vi "Main_PhaseShifting.vi"() -> ()   [LabVIEW 2020]
uses:
  Controls/Control_Camara.ctl
  <vilib>/userdefined/High Color/IMAQdx.ctl
  Controls/Control_MaquinaEstados.ctl
  Controls/Control_RegistroDeDatos.ctl
  <vilib>/vision/Image Controls.llb/IMAQ Image.ctl
  <vilib>/Instr/_visa.llb/VISA Find Search Mode.ctl
  <vilib>/Instr/_visa.llb/VISA Configure Serial Port (Instr).vi
  <vilib>/vision/driver/NI_Vision_Acquisition_Software.lvlib
panel:
  in  "Session In":T1
  out "InterfaceName":string
  in  "Numero de Pasos":i32=5
  in  "Delay piezoeléctrico (ms)":u32=500
  in  "Nombre de la Imagen":string="Referencia"
  out "Voltaje Enviado":string[](array[string])
  in  "SnapShot":bool
  out "Pantalla":T2(plugin-control)
  in  "Puerto":refnum<visa-resource-name>="COM2"
  in  "Fotos":T3
  in  "Calibrar":bool
  in  "stop":bool
  # "#TODO: add selector for manual/auto phase shifting."
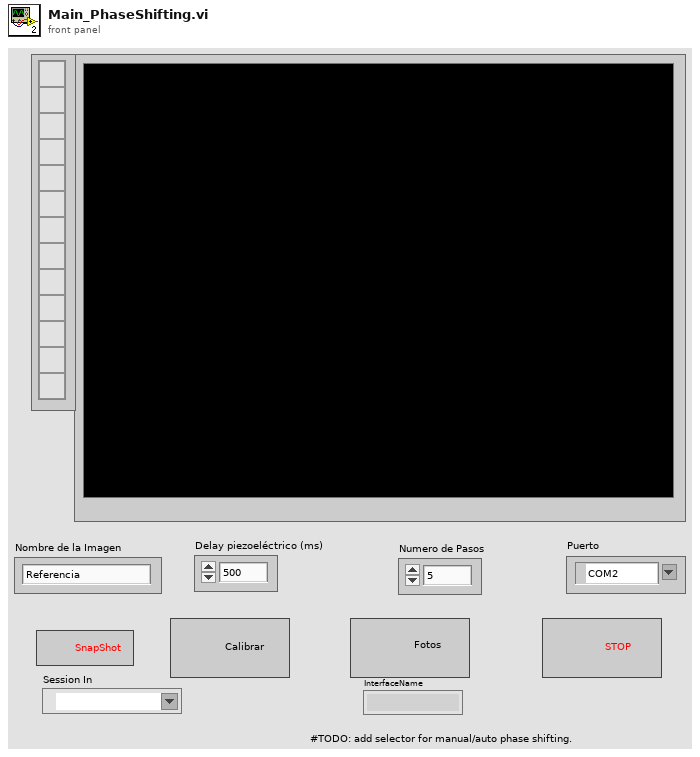
[diagram p1: front panel]
types:
  T1 = typedef "IMAQdx.ctl" = refnum<k21>
  T2 = typedef "IMAQ Image.ctl" = refnum<image>
  T3 = typedef "Control_Camara.ctl" = bool
  T4 = typedef "Control_RegistroDeDatos.ctl" = cluster{"V 2Pi Actual":sgl, "Puerto":refnum<visa-resource-name>, "InterfaceName":string, "Canal":string, "dt (ms)":u16, "Referencias":cluster{"Calibrar":refnum<vi>, "Fotos":refnum<vi>, "stop":refnum<vi>, "SnapShot":refnum<vi>}, "Imagenes":T2[], "Session Out":T1, "Bandera":bool}
  T5 = typedef "Control_MaquinaEstados.ctl" = enum16{"Esperar", "Inicializar", "Calibración", "Fotos", "Grabando", "Inicializar dispositivos", "Fase", "Cerrar dispositivos", "Exit"}
  T6 = typedef "VISA Find Search Mode.ctl" = u32
  T7 = cluster{"Type":u32, "Version":u32, "Flags":u32, "SerialNumberHigh":u32, "SerialNumberLow":u32, "BusType":u32, "InterfaceName":string, "VendorName":string, "ModelName":string, "CameraFileName":string, "CameraAttributeURL":string}[]
  T8 = cluster{"Type":u32, "Version":u32, "Flags":u32, "SerialNumberHigh":u32, "SerialNumberLow":u32, "BusType":u32, "InterfaceName":string, "VendorName":string, "ModelName":string, "CameraFileName":string, "CameraAttributeURL":string}
  T9 = cluster{"Calibrar":refnum<vi>, "Fotos":refnum<vi>, "stop":refnum<vi>, "SnapShot":refnum<vi>}
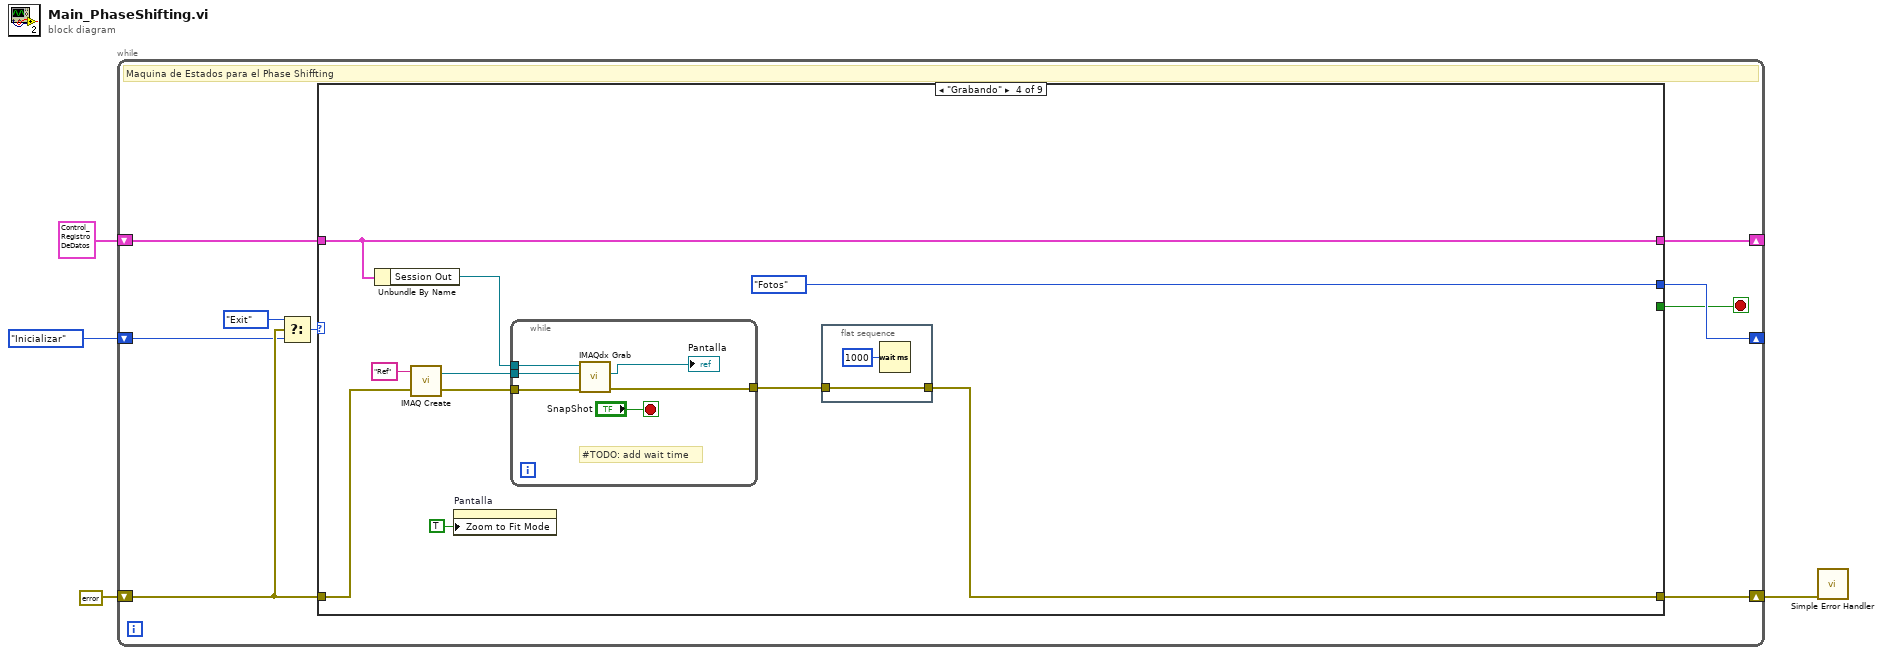
[diagram p0: block diagram]
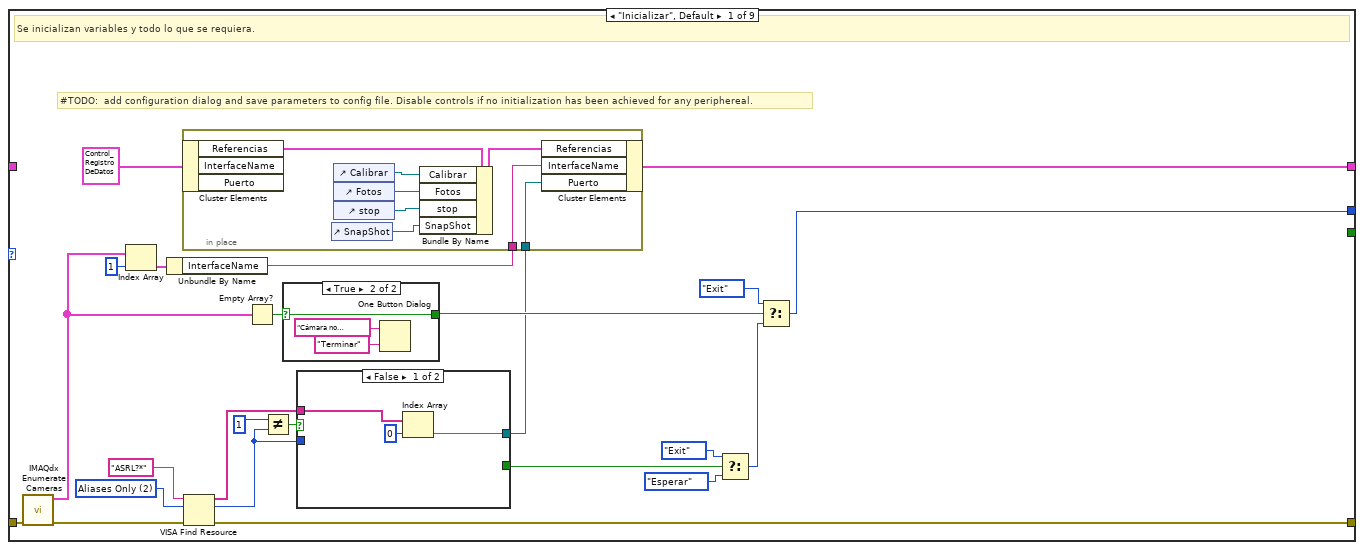
[diagram p2: hidden frame]
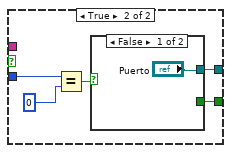
[diagram p3: hidden frame]
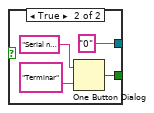
[diagram p4: hidden frame]
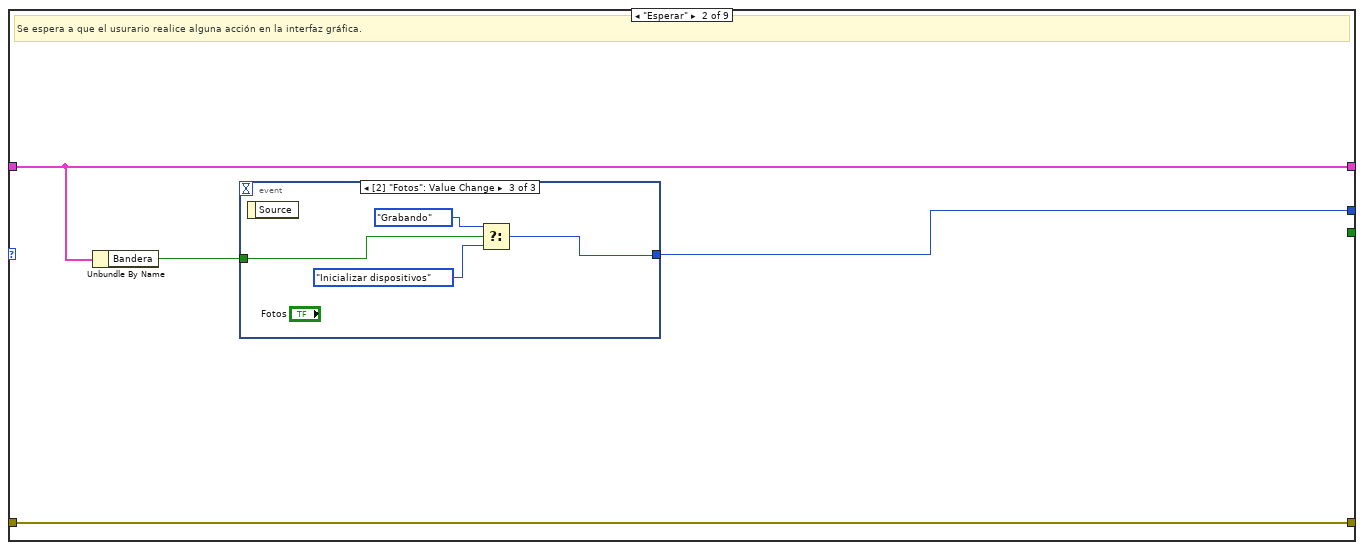
[diagram p6: hidden frame]
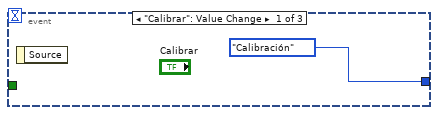
[diagram p7: hidden frame]
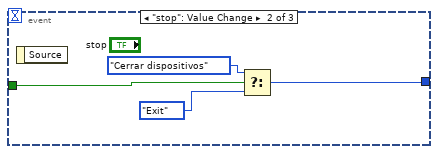
[diagram p8: hidden frame]
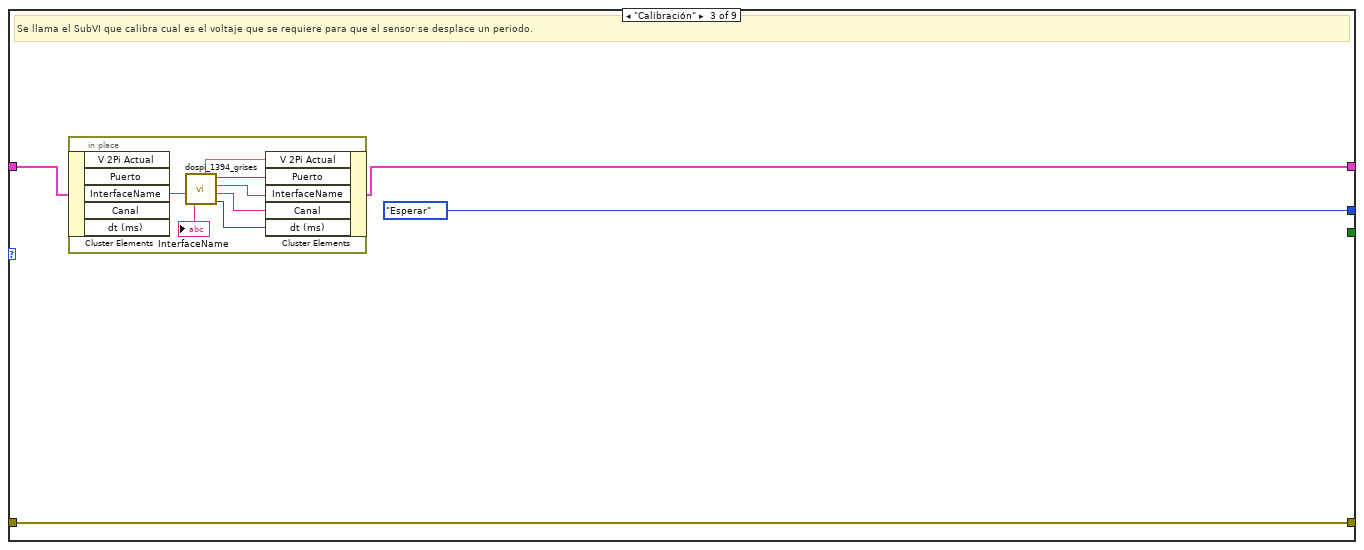
[diagram p9: hidden frame]
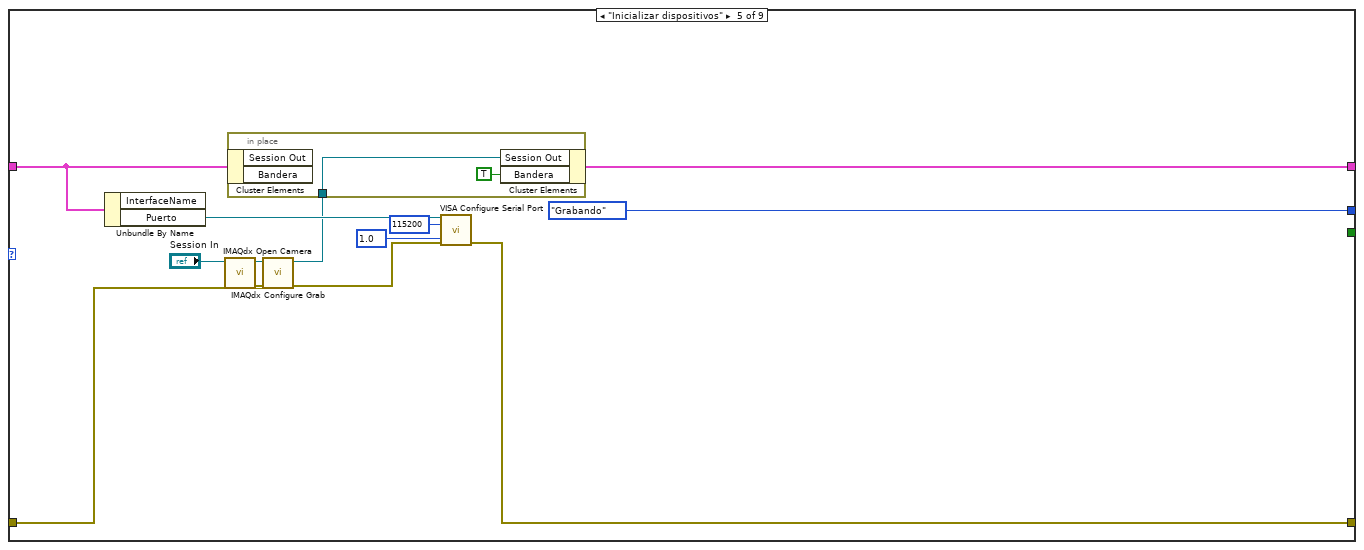
[diagram p10: hidden frame]
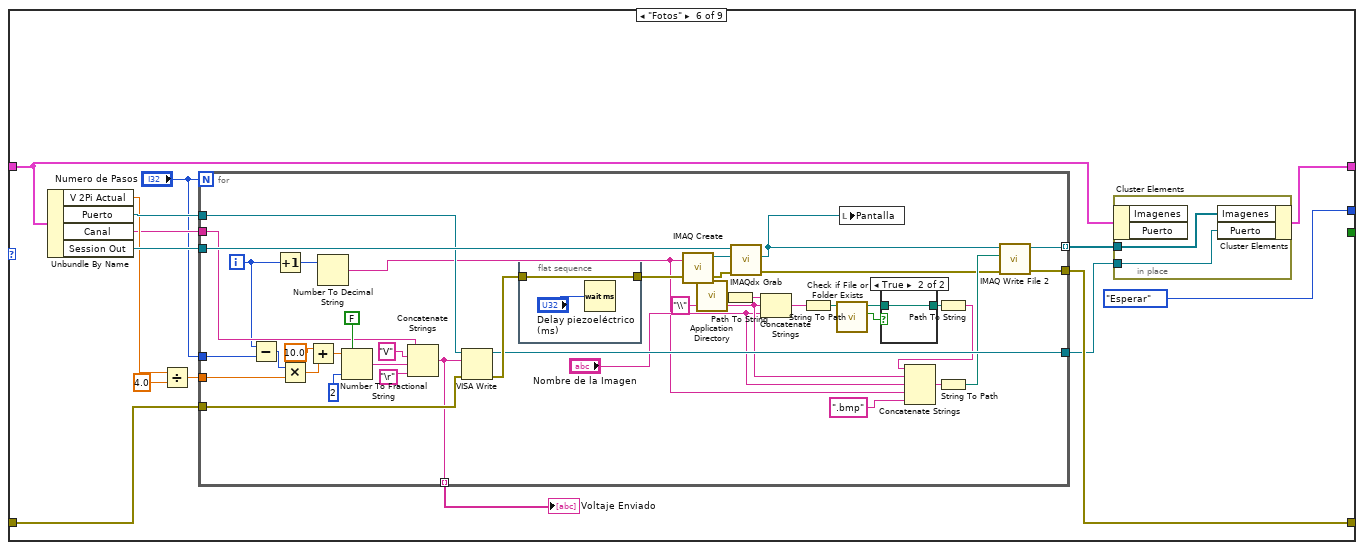
[diagram p11: hidden frame]
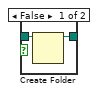
[diagram p12: hidden frame]
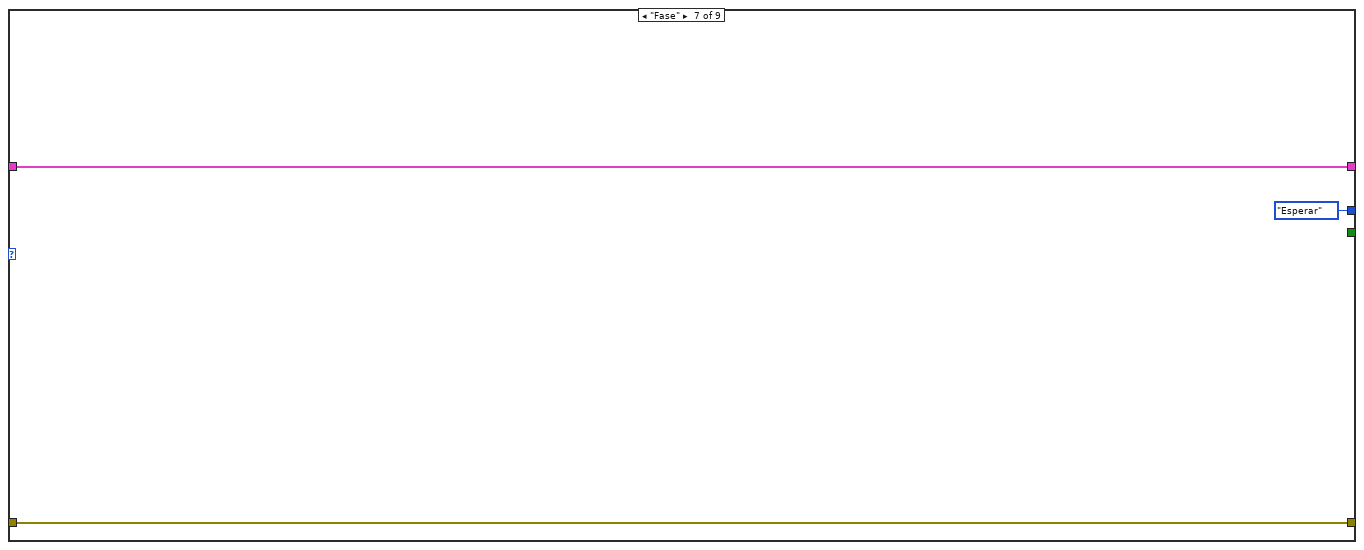
[diagram p13: hidden frame]
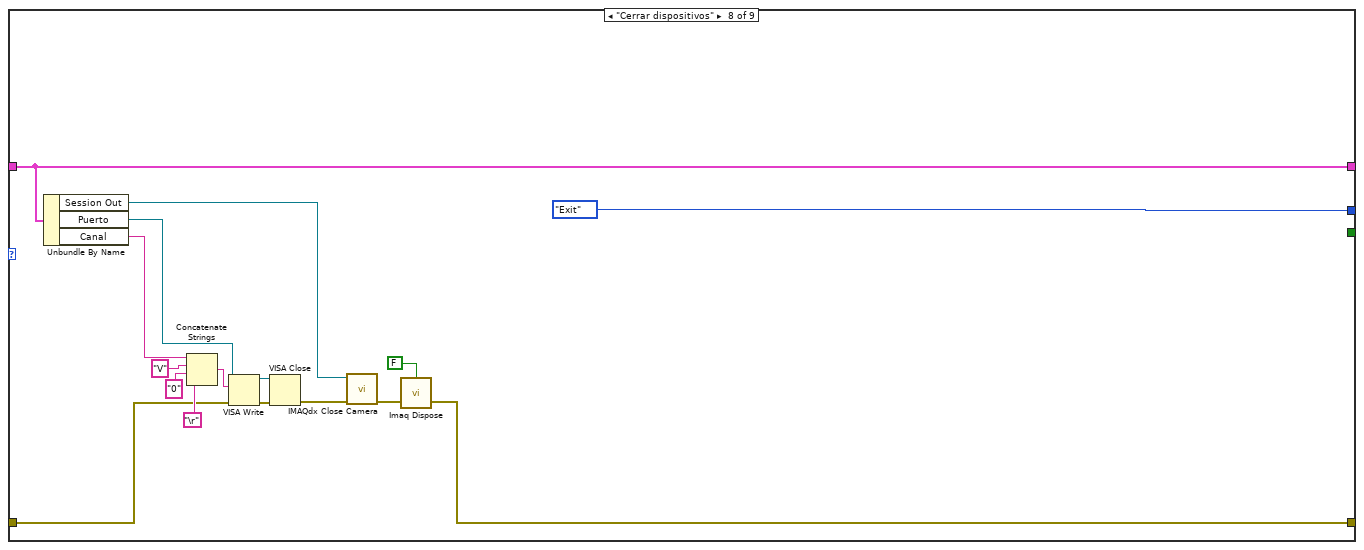
[diagram p14: hidden frame]
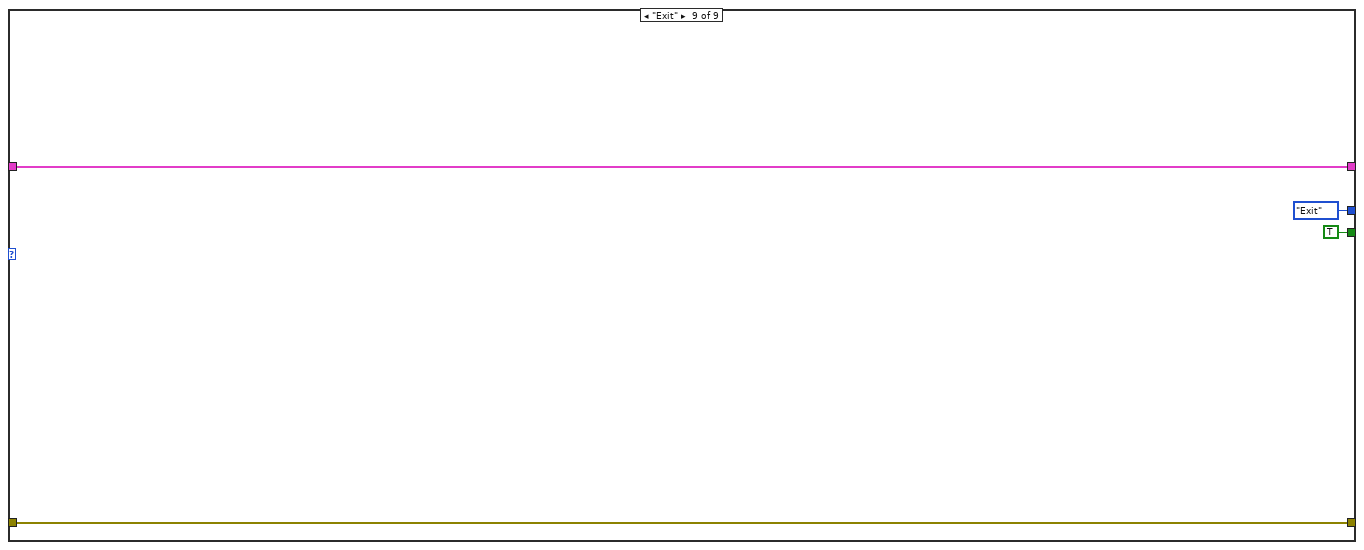
[diagram p15: hidden frame]
diagram:
  n1 = while {
    shift-right: [w13] -> _
    shift-left: Control_MaquinaEstados."Inicializar" ("Enum") -> [w10]
    shift-right: [w12] -> _
    shift-left: T4 {"V 2Pi Actual"=0.0, "Puerto"="COM3", "InterfaceName"="", "Canal"="", "dt (ms)"=0, "Referencias"={"Calibrar"=refnum, "Fotos"=refnum, "stop"=refnum, "SnapShot"=refnum}, "Imagenes"=[], "Session Out"="cam11", "Bandera"=FALSE} -> [w5]
    shift-right: [w6] -> w3
    shift-left: errorcluster {"status"=FALSE, "code"=0, "source"=""} ("Error In") -> [w11]
    stop <- w7 stop-if-true
    # "Maquina de Estados para el Phase Shiffting"
    n2 = Select(t=Control_MaquinaEstados."Exit", s=w11, f=w10) -> (s? t:f=w8:T5)
    n3 = case shown="\"Grabando\"" w8 {
      tunnel: [w19 w66 Control_MaquinaEstados."Esperar" ("Enum") Control_MaquinaEstados."Fotos" ("Enum") Control_MaquinaEstados."Grabando" ("Enum") Control_MaquinaEstados."Esperar" ("Enum") Control_MaquinaEstados."Esperar" ("Enum") Control_MaquinaEstados."Exit" ("Enum") Control_MaquinaEstados."Exit" ("Enum")] -> w13
      tunnel: w5 -> [_ w64 w79 w88 w107 w126 w184 w193 w204]
      tunnel: [w37 w64 w78 w88 w105 w123 w184 w193 w204] -> w12
      tunnel: [_ _ _ _ _ _ _ _ TRUE] -> w7
      tunnel: w11 -> [w17 w65 w76 w94 w109 w132 w183 w190 w203]
      tunnel: [w15 w65 w76 w89 w112 w131 w183 w185 w203] -> w6
      frame "Inicializar", Default {
        w31 = T6 2 items=["Canonical Names Only"=0, "Aliases Only"=2, "Include Matching Aliases"=3, "Include All Aliases"=4] ("Search Mode")
        # "#TODO:  add configuration dialog and save parameters to config file. Disable controls if no initialization has been achieved for any periphereal."
        # "Se inicializan variables y todo lo que se requiera."
        n4 = call <vilib>:"IMAQdx Enumerate Cameras.vi"("error in"=w17) -> ("error out"=w16:errorcluster, "Camera Information Array"=w29:T7)  [unwired: 9 in]
        n5 = Index Array(array=w29, index=1) -> (element=w28:T8)
        n6 = Unbundle By Name(w28) -> ("InterfaceName"=w26:string)
        n7 = VISA Find Resource(8:w16, 10:w31, 11:"ASRL?*" ("expression (\"?*\")")) -> (0:w15:errorcluster, 2:w35:u32, 3:w34:string[])
        n8 = Empty Array?(array=w29) -> (empty?=w30:bool)
        n9 = Not Equal?(x=u32 1 ("y"), y=w35) -> (x != y?=w33:bool)
        n10 = case shown="True" w30 {
          selector: w30 -> [w51 w52]
          tunnel: [w51 w52] -> w25
          frame False {
          }
          frame True {
            n11 = One Button Dialog(message="Cámara no encontrada" ("error source (\" \")"), button name ("OK")="Terminar") -> ()  [unwired: 1 out]
          }
        }
        n12 = case shown="False" w33 {
          tunnel: w34 -> [w40 _]
          tunnel: [w38 w45] -> w18
          tunnel: w35 -> [_ w44]
          tunnel: [_ w42] -> w24
          frame False {
            n13 = Index Array(array=w40, index=0) -> (element=w38:string)
          }
          frame True {
            n14 = Equal?(x=w44, y=u32 0) -> (x = y?=w43:bool)
            n15 = case shown="False" w43 {
              tunnel: ["Puerto" "0" ("button name (\"OK\")")] -> w45
              tunnel: [_ w48] -> w42
              frame False {
              }
              frame True {
                n16 = One Button Dialog(message="Serial no encontrado" ("error source (\" \")"), button name ("OK")="Terminar") -> (true=w48:bool)
              }
            }
          }
        }
        n17 = in-place {
          in-place-border: w26 -> [w57]
          in-place-border: w18 -> [w56]
          n18 = in-place-cluster #1(T4 {"V 2Pi Actual"=0.0, "Puerto"="COM3", "InterfaceName"="", "Canal"="", "dt (ms)"=0, "Referencias"={"Calibrar"=refnum, "Fotos"=refnum, "stop"=refnum, "SnapShot"=refnum}, "Imagenes"=[], "Session Out"="cam11", "Bandera"=FALSE}) -> ("Referencias"=w62:T9)  [unwired: 2 out]
          n19 = control-ref of="SnapShot"() -> (w55:refnum<vi>)
          n20 = control-ref of="Calibrar"() -> (w60:refnum<vi>)
          n21 = control-ref of="Fotos"() -> (w59:refnum<vi>)
          n22 = control-ref of="stop"() -> (w58:refnum<vi>)
          n23 = Bundle By Name(cluster=w62, "Calibrar"=w60, "Fotos"=w59, "stop"=w58, "SnapShot"=w55) -> (w61:T9)
          n24 = in-place-cluster #1("Referencias"=w61, "InterfaceName"=w57, "Puerto"=w56) -> (w37:T4)
        }
        n25 = Select(t=Control_MaquinaEstados."Exit" ("Enum"), s=w24, f=Control_MaquinaEstados."Esperar" ("Enum")) -> (s? t:f=w21:T5)
        n26 = Select(t=Control_MaquinaEstados."Exit" ("Enum"), s=w25, f=w21) -> (s? t:f=w19:T5)
      }
      frame "Esperar" {
        # "Se espera a que el usurario realice alguna acción en la interfaz gráfica."
        n27 = Unbundle By Name(w64) -> ("Bandera"=w63:bool)
        n28 = event shown="[2] \"Fotos\": Value Change" {
          selector: _ -> [_ _ _]
          dyn-events: _ -> [_ _ _]
          timeout: _ -> [_ _ _]
          tunnel: [Control_MaquinaEstados."Calibración" ("Enum") w68 w73] -> w66
          tunnel: w63 -> [_ w71 w75]
          event "Calibrar": Value Change {
            n29 = event-data() -> ()  [unwired: 1 in, 1 out]
          }
          event "stop": Value Change {
            n30 = event-data() -> ()  [unwired: 1 in, 1 out]
            n31 = Select(t=Control_MaquinaEstados."Cerrar dispositivos" ("Enum"), s=w71, f=Control_MaquinaEstados."Exit" ("Enum")) -> (s? t:f=w68:T5)
          }
          event Value Change {
            n32 = event-data() -> ()  [unwired: 1 in, 1 out]
            n33 = Select(t=Control_MaquinaEstados."Grabando" ("Enum"), s=w75, f=Control_MaquinaEstados."Inicializar dispositivos" ("Enum")) -> (s? t:f=w73:T5)
          }
        }
      }
      frame "Calibración" {
        # "Se llama el SubVI que calibra cual es el voltaje que se requiere para que el sensor se desplace un periodo."
        n34 = in-place {
          n35 = in-place-cluster #2(w79) -> ("InterfaceName"=→"InterfaceName":string)  [unwired: 4 out]
          n36 = call "dospi_1394_grises.vi"() -> ("dt (ms) 2"=w81:u16, "Canal 2"=w82:string, "InterfaceName"=w83:string, "Puerto 2"=w84:refnum<visa-resource-name>, "V 2Pi\nActual"=w85:sgl)  [unwired: 6 in, 1 out]
          n37 = in-place-cluster #2("V 2Pi Actual"=w85, "Puerto"=w84, "InterfaceName"=w83, "Canal"=w82, "dt (ms)"=w81) -> (w78:T4)
        }
      }
      frame "Grabando" {
        n38 = Unbundle By Name(w88) -> ("Session Out"=w87:T1)
        n39 = call "IMAQ Create"("Image Name"="Ref", "error in (no error)"=w94) -> ("New Image"=w93:T2, "error out"=w91:errorcluster)  [unwired: 3 in]
        n40 = property on="Pantalla" class="ImageControl"("Zoom to Fit Mode"=TRUE) -> ()  [unwired: 2 in, 2 out]
        n41 = while {
          tunnel: w87 -> [w103]
          tunnel: w91 -> [w102]
          tunnel: w93 -> [w101]
          tunnel: [w98] -> w90
          stop <- "SnapShot" stop-if-true
          # "#TODO: add wait time"
          n42 = call <vilib>:"IMAQdx Grab.vi"("error in"=w102, "Image In"=w101, "Session In"=w103) -> ("error out"=w98:errorcluster, "Image Out"=→"Pantalla":T2)  [unwired: 5 in, 2 out]
        }
        n43 = flat-sequence {
          tunnel: w90 -> [w96]
          tunnel: [w96] -> w89
          frame #0 {
            n44 = Wait (ms)(milliseconds to wait=u32 1000) -> ()  [unwired: 1 out]
          }
        }
      }
      frame "Inicializar dispositivos" {
        w114 = u16 10 items=["1.0"=10, "1.5"=15, "2.0"=20] ("stop bits (10: 1 bit)")
        n45 = Unbundle By Name(w107) -> ("Puerto"=w111:refnum<visa-resource-name>)  [unwired: 1 out]
        n46 = call <vilib>:"IMAQdx Open Camera.vi"("error in"=w109, "Session In"="Session In") -> ("error out"=w115:errorcluster, "Session Out"=w116:T1)  [unwired: 8 in]
        n47 = call <vilib>:"IMAQdx Configure Grab.vi"("error in"=w115, "Session In"=w116) -> ("error out"=w108:errorcluster, "Session Out"=w106:T1)  [unwired: 8 in]
        n48 = in-place {
          in-place-border: w106 -> [w118]
          n49 = in-place-cluster #3(w107) -> ()  [unwired: 2 out]
          n50 = in-place-cluster #3("Session Out"=w118, "Bandera"=TRUE) -> (w105:T4)
        }
        n51 = call-poly "VISA Configure Serial Port"("VISA resource name"=w111, "baud rate (9600)"=u32 115200, "error in (no error)"=w108, "stop bits (10: 1 bit)"=w114) -> ("error out"=w112:errorcluster)  [unwired: 10 in, 1 out]
      }
      frame "Fotos" {
        n52 = Unbundle By Name(w126) -> ("V 2Pi Actual"=w129:sgl, "Puerto"=w130:refnum<visa-resource-name>, "Canal"=w127:string, "Session Out"=w133:T1)
        n53 = Divide(x=w129, y=sgl 4.0) -> (x/y=w128:sgl)
        n54 = for {
          N: "Numero de Pasos" -> [_]
          tunnel: w133 -> [w176]
          tunnel: w132 -> [w160]
          tunnel: [w153] -> w125 mode=indexing
          tunnel: [w154] -> w131
          tunnel: w130 -> [w165]
          tunnel: w128 -> [w161]
          tunnel: w127 -> [w164]
          tunnel: [w156] -> w124
          tunnel: [w155] -> w120 mode=indexing
          tunnel: "Numero de Pasos" -> [w136]
          i -> [w162]
          w143 = "\\" ("string")
          n55 = Subtract(x=w162, y=w136) -> (x-y=w163:i32)
          n56 = Increment(x=w162) -> (x+1=w175:i32)
          n57 = Multiply(x=w163, y=w161) -> (x*y=w166:sgl)
          n58 = Add(x=sgl 10.0, y=w166) -> (x+y=w173:sgl)
          n59 = Number To Decimal String(number=w175) -> (decimal integer string=w141:string)  [unwired: 1 in]
          n60 = Number To Fractional String(use system decimal point (T)=FALSE, number=w173, precision (6)=i16 2) -> (F-format string=w167:string)  [unwired: 1 in]
          n61 = Concatenate Strings(w164, "V" ("Substring"), w167, "\r") -> (w155:string)
          n62 = VISA Write(VISA resource name=w165, write buffer=w155, error in (no error)=w160) -> (VISA resource name out=w156:refnum<visa-resource-name>, error out=w158:errorcluster)  [unwired: 1 out]
          n63 = flat-sequence {
            tunnel: w158 -> [w180]
            tunnel: [w180] -> w157
            frame #0 {
              n64 = Wait (ms)(milliseconds to wait="Delay piezoeléctrico (ms)") -> ()  [unwired: 1 out]
            }
          }
          n65 = call "IMAQ Create"("Image Name"=w141, "error in (no error)"=w157) -> ("New Image"=w174:T2, "error out"=w159:errorcluster)  [unwired: 3 in]
          n66 = call <vilib>:"Application Directory.vi"() -> ("Application Directory"=w152:path)
          n67 = Path To String(path=w152) -> (string=w151:string)
          n68 = call <vilib>:"IMAQdx Grab.vi"("error in"=w159, "Image In"=w174, "Session In"=w176) -> ("error out"=w138:errorcluster, "Image Out"=w137:T2)  [unwired: 5 in, 2 out]
          n69 = Concatenate Strings(w151, w143, "Nombre de la Imagen") -> (w150:string)
          n70 = String To Path(string=w150) -> (path=w147:path)
          n71 = call <vilib>:"Check if File or Folder Exists.vi"("path"=w147) -> ("file or folder exists?"=w148:bool, "dup path"=w149:path)  [unwired: 8 in, 1 out]
          n72 = local write "Pantalla"(w137) -> ()
          n73 = case shown="True" w148 {
            tunnel: w149 -> [w178 w179]
            tunnel: [w177 w179] -> w145
            frame False {
              n74 = Create Folder(path (use dialog)=w178) -> (created path=w177:path)  [unwired: 2 in, 2 out]
            }
            frame True {
            }
          }
          n75 = Path To String(path=w145) -> (string=w144:string)
          n76 = Concatenate Strings(w144, w143, "Nombre de la Imagen", w141, ".bmp" ("string")) -> (w146:string)
          n77 = String To Path(string=w146) -> (path=w139:path)
          n78 = call-poly "IMAQ Write File 2"("error in (no error)"=w138, "File Path"=w139, "Image"=w137) -> ("error out"=w154:errorcluster, "Image Out (duplicate)"=w153:T2)  [unwired: 7 in]
        }
        "Voltaje Enviado" <- w120
        n79 = in-place {
          in-place-border: w125 -> [w134]
          in-place-border: w124 -> [w135]
          n80 = in-place-cluster #4(w126) -> ()  [unwired: 2 out]
          n81 = in-place-cluster #4("Imagenes"=w134, "Puerto"=w135) -> (w123:T4)
        }
      }
      frame "Fase" {
      }
      frame "Cerrar dispositivos" {
        n82 = Unbundle By Name(w193) -> ("Session Out"=w188:T1, "Puerto"=w192:refnum<visa-resource-name>, "Canal"=w191:string)
        n83 = Concatenate Strings(w191, "V" ("Substring"), "0" ("Substring"), "\r") -> (w196:string)
        n84 = VISA Write(VISA resource name=w192, write buffer=w196, error in (no error)=w190) -> (VISA resource name out=w194:refnum<visa-resource-name>, error out=w195:errorcluster)  [unwired: 1 out]
        n85 = VISA Close(VISA resource name=w194, error in (no error)=w195) -> (error out=w187:errorcluster)
        n86 = call <vilib>:"IMAQdx Close Camera.vi"("error in"=w187, "Session In"=w188) -> ("error out"=w186:errorcluster)  [unwired: 9 in]
        n87 = call "Imaq Dispose"("All Images? (No)"=FALSE, "error in (no error)"=w186) -> ("error out"=w185:errorcluster)  [unwired: 4 in]
      }
      frame "Exit" {
      }
    }
  }
  n88 = call <vilib>:"Simple Error Handler.vi"("error in (no error)"=w3) -> ()  [unwired: 4 in, 5 out]
